vi "Wind Power Array.vi"(9 "Wind Speed (m/s)":dbl[](array[numeric]), 10 "Density (kg/m^3)":dbl, 11 "Blade Length (m)":dbl) -> (1 "Power (watts)":dbl[](array[numeric]))   [LabVIEW 2018]
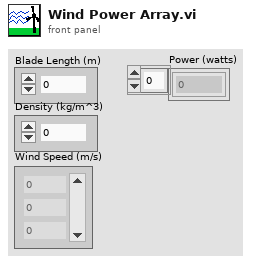
[diagram p1: front panel]
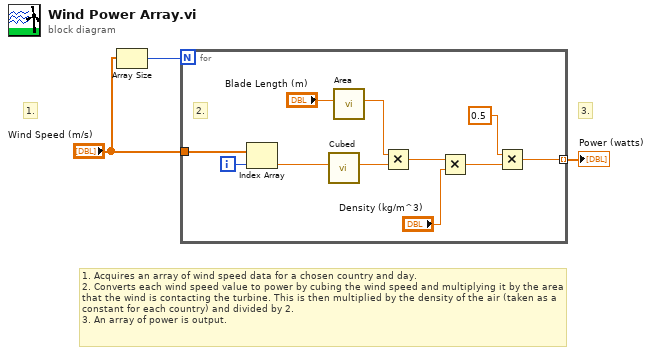
[diagram p0: block diagram]
diagram:
  # "3."
  # "1."
  # "1. Acquires an array of wind speed data for a chosen country and day.\n2. Converts each wind speed value to power by cubing the wind speed and multiplying it by the area that the wind is contacting the turbine. This is then multiplied by the density of the air (taken as a constant for each country) and divided by 2.\n3. An array of power is output."
  n1 = Array Size(array="Wind Speed (m/s)") -> (size(s)=w1:i32)
  n2 = for {
    N: w1 -> [_]
    tunnel: [w7] -> w3 mode=indexing
    tunnel: "Wind Speed (m/s)" -> [w5]
    i -> [w6]
    # "2."
    n3 = Index Array "Index Array"(array=w5, index=w6) -> (element=w4:dbl)
    n4 = call "Cubed.vi"("X"=w4) -> ("X^3"=w13:dbl)  [unwired: 10 in]
    n5 = call "Area.vi"("Blade Length (m/s)"="Blade Length (m)") -> ("Area (m^2)"=w12:dbl)  [unwired: 10 in]
    n6 = Multiply(x=w12, y=w13) -> (x*y=w10:dbl)
    n7 = Multiply(x=w10, y="Density (kg/m^3)") -> (x*y=w9:dbl)
    n8 = Multiply(x=0.5, y=w9) -> (x*y=w7:dbl)
  }
  "Power (watts)" <- w3
